vi "runReceiver.vi"(8 "error in (no error)":errorcluster, 10 "ScriptEvent":refnum<class "ScriptEvent.lvclass">, 11 "receiver in":refnum<class "receiver.lvclass">) -> (0 "error out":errorcluster, 3 "receiver out":refnum<class "receiver.lvclass">)   [LabVIEW 2011, in "Events.lvlib" / "receiver.lvclass"]
uses:
  receiver.lvclass
  ScriptEvent.lvclass
  Event.lvclass
panel:
  in  "saveUnregister":bool=TRUE
  out "Path":path
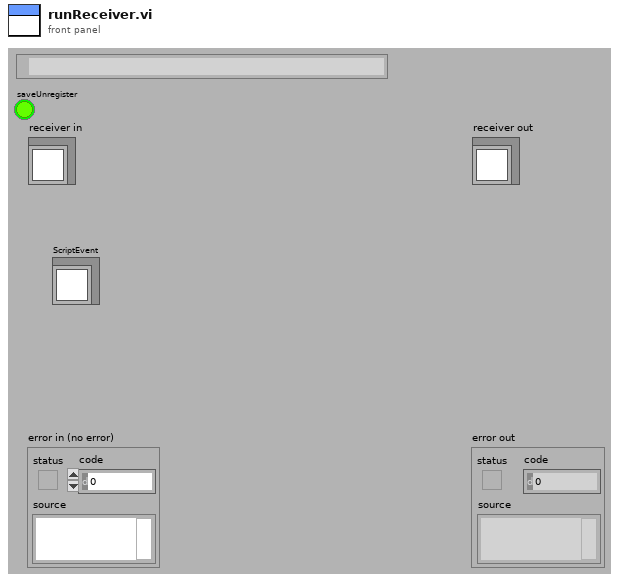
[diagram p1: front panel]
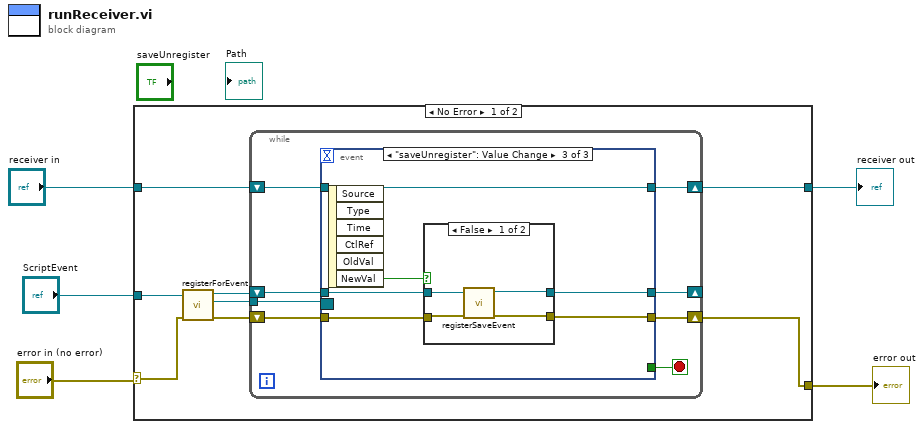
[diagram p0: block diagram]
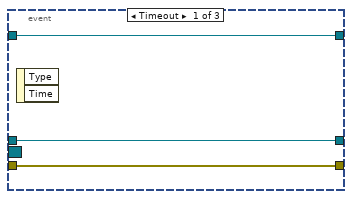
[diagram p2: hidden frame]
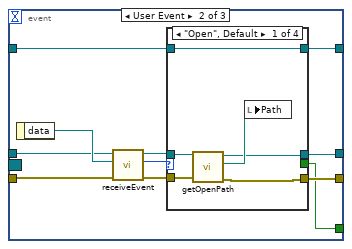
[diagram p3: hidden frame]
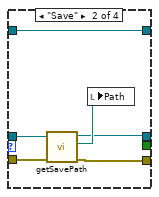
[diagram p4: hidden frame]
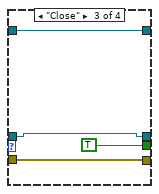
[diagram p5: hidden frame]
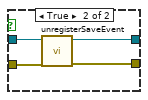
[diagram p7: hidden frame]
diagram:
  n1 = case shown="No Error" "error in (no error)" {
    selector: "error in (no error)" -> [w10 w70]
    tunnel: [w7 w70] -> w4
    tunnel: [w12 w69] -> w2
    tunnel: "receiver in" -> [w13 w69]
    tunnel: "ScriptEvent" -> [w11 _]
    frame No Error {
      n2 = call "registerForEvent.vi"("error in (no error)"=w10, "Event in"=w11) -> ("error out"=w8:errorcluster, "Event Registration Refnum"=w9:refnum<event-registration>, "Event out"=w6:refnum<class "ScriptEvent.lvclass">)  [unwired: 6 in, 1 out]
      n3 = while {
        shift-right: [w20] -> w12
        shift-left: w13 -> [w21]
        tunnel: w9 -> [w19]
        shift-right: [w17] -> w7
        shift-left: w8 -> [w18]
        shift-right: [w15] -> _
        shift-left: w6 -> [w14]
        stop <- w16 stop-if-true
        n4 = event shown="[2] \"saveUnregister\": Value Change" {
          selector: w19 -> [_ _ _]
          dyn-events: _ -> [_ _ _]
          timeout: _ -> [_ _ _]
          tunnel: w21 -> [w24 w27 w60]
          tunnel: [w24 w26 w60] -> w20
          tunnel: w18 -> [w23 w33 w58]
          tunnel: [w23 w29 w56] -> w17
          tunnel: w14 -> [w22 w34 w59]
          tunnel: [_ w28 _] -> w16
          tunnel: [w22 w25 w55] -> w15
          event Timeout {
            n5 = event-data() -> ()  [unwired: 1 in, 2 out]
          }
          event User Event {
            n6 = event-data() -> ("data"=w35:refnum<class>)  [unwired: 1 in]
            n7 = call "receiveEvent.vi"("error in (no error)"=w33, "data"=w35, "ScriptEvent in"=w34) -> ("error out"=w30:errorcluster, "Event Type"=w32:enum16{"Open", "Save", "Close", "Unregistered"}, "ScriptEvent out"=w31:refnum<class "ScriptEvent.lvclass">)  [unwired: 6 in]
            n8 = case shown="\"Open\", Default" w32 {
              tunnel: w31 -> [w41 w47 w48 w52]
              tunnel: w30 -> [w40 w46 w51 w54]
              tunnel: [w38 w44 w51 w54] -> w29
              tunnel: [_ _ TRUE _] -> w28
              tunnel: w27 -> [w37 w43 w49 w53]
              tunnel: [w37 w43 w49 w53] -> w26
              tunnel: [w36 w42 w48 w52] -> w25
              frame "Open", Default {
                n9 = call "getOpenPath.vi"("error in (no error)"=w40, "ScriptEvent in"=w41) -> ("error out"=w38:errorcluster, "openPath"=w39:path, "ScriptEvent out"=w36:refnum<class "ScriptEvent.lvclass">)  [unwired: 7 in]
                n10 = local write "Path"(w39) -> ()
              }
              frame "Save" {
                n11 = call "getSavePath.vi"("error in (no error)"=w46, "ScriptEvent in"=w47) -> ("error out"=w44:errorcluster, "savePath"=w45:path, "ScriptEvent out"=w42:refnum<class "ScriptEvent.lvclass">)  [unwired: 7 in]
                n12 = local write "Path"(w45) -> ()
              }
              frame "Close" {
              }
              frame "Unregistered" {
              }
            }
          }
          event "saveUnregister": Value Change {
            n13 = event-data() -> ("NewVal"=w57:bool)  [unwired: 1 in, 5 out]
            n14 = case shown="False" w57 {
              tunnel: w59 -> [w64 w68]
              tunnel: w58 -> [w61 w67]
              tunnel: [w62 w66] -> w56
              tunnel: [w63 w65] -> w55
              frame False {
                n15 = call "registerSaveEvent.vi"("error in (no error)"=w61, "ScriptEvent in"=w64) -> ("error out"=w62:errorcluster, "ScriptEvent out"=w63:refnum<class "ScriptEvent.lvclass">)  [unwired: 8 in]
              }
              frame True {
                n16 = call "unregisterSaveEvent.vi"("error in (no error)"=w67, "ScriptEvent in"=w68) -> ("error out"=w66:errorcluster, "ScriptEvent out"=w65:refnum<class "ScriptEvent.lvclass">)  [unwired: 8 in]
              }
            }
          }
        }
      }
    }
    frame Error {
    }
  }
  "error out" <- w4
  "receiver out" <- w2
